vi "EMS Setpoint Status.vi"(4 "Status":T1, 6 "Error String":string, 8 "error in (no error)":errorcluster, 9 "Variable Name":string, 10 "IED Name":string, 11 "Master Controller in":refnum<class "Master Controller.lvclass">) -> (0 "error out":errorcluster, 3 "Master Controller out":refnum<class "Master Controller.lvclass">)   [LabVIEW 2015, in "Master Controller Core.lvlib" / "Master Controller.lvclass"]
uses:
  Master Controller.lvclass
  SCADA Core/SCADA Abstract Messages/IED Setpoint Status Msg/IED Setpoint Status.ctl
  Communications/SCADA Communcations Actor/SCADA Communications/Controls/EMS Message Cluster.ctl
  Master Controller.lvclass/Master Controller.ctl
  Communications/SCADA Communcations Actor/SCADA Communications Messages/Transmit EMS Message Msg/Transmit EMS Message Msg.lvclass/Transmit EMS Message Msg.ctl
  <vilib>/ActorFramework/Message Enqueuer/Message Enqueuer.lvclass/Message Enqueuer.ctl
  <vilib>/ActorFramework/Message Enqueuer/Enqueue.vi
  <vilib>/ActorFramework/Message Priority Queue/Priority Enqueue.vi
  Communications/SCADA Communcations Actor/SCADA Communications Messages/Transmit EMS Message Msg/Transmit EMS Message Msg.lvclass
  Utilities/Message Strings.llb/Message String Utilities.lvlib
  Communications/SCADA Communcations Actor/SCADA Communications/SCADA Communications.lvclass
  SCADA Core/SCADA Abstract Messages/IED Setpoint Status Msg/IED Setpoint Status Msg.lvclass
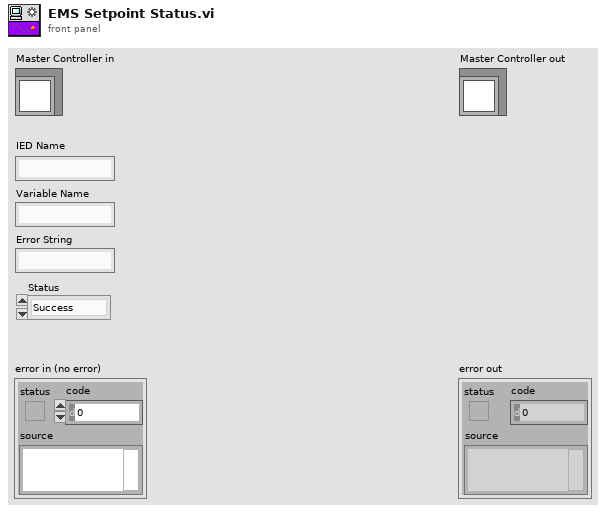
[diagram p1: front panel]
types:
  T1 = typedef "SCADA Core.lvlib/IED Setpoint Status Msg.lvclass/IED Setpoint Status.ctl" = enum16{"Success", "Failure", "Multiple Success", "Multiple Failure"}
  T2 = typedef "SCADA Communcations Actor.lvlib/SCADA Communications.lvclass/EMS Message Cluster.ctl" = cluster{"Name":string, "Content":string}
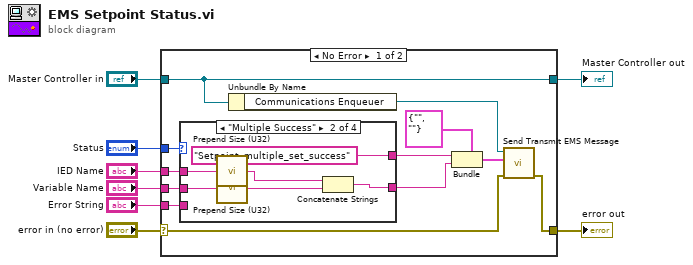
[diagram p0: block diagram]
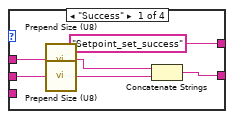
[diagram p2: hidden frame]
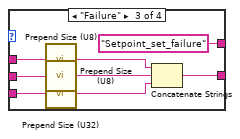
[diagram p3: hidden frame]
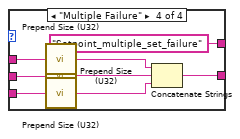
[diagram p4: hidden frame]
diagram:
  n1 = case shown="No Error" "error in (no error)" {
    selector: "error in (no error)" -> [w14 w50]
    tunnel: [w9 w50] -> w7
    tunnel: [w15 w49] -> w5
    tunnel: "Master Controller in" -> [w15 w49]
    tunnel: "Status" -> [w13 _]
    tunnel: "IED Name" -> [w12 _]
    tunnel: "Variable Name" -> [w11 _]
    tunnel: "Error String" -> [w10 _]
    frame No Error {
      n2 = case shown="\"Multiple Success\"" w13 {
        tunnel: ["Setpoint_set_success" ("Name") "Setpoint_multiple_set_success" ("Name") "Setpoint_set_failure" ("Name") "Setpoint_multiple_set_failure" ("Name")] -> w19
        tunnel: w10 -> [_ _ w38 w46]
        tunnel: w11 -> [w25 w31 w39 w47]
        tunnel: w12 -> [w24 w30 w37 w45]
        tunnel: [w21 w27 w33 w41] -> w20
        frame "Success" {
          n3 = call "Prepend Size (U8).vi"("String in"=w24) -> ("String out"=w23:string)
          n4 = call "Prepend Size (U8).vi"("String in"=w25) -> ("String out"=w22:string)
          n5 = Concatenate Strings(w23, w22) -> (w21:string)
        }
        frame "Multiple Success" {
          n6 = call "Prepend Size (U32).vi"("String in"=w30) -> ("String out"=w29:string)
          n7 = call "Prepend Size (U32).vi"("String in"=w31) -> ("String out"=w28:string)
          n8 = Concatenate Strings(w29, w28) -> (w27:string)
        }
        frame "Failure" {
          n9 = call "Prepend Size (U8).vi"("String in"=w37) -> ("String out"=w35:string)
          n10 = call "Prepend Size (U8).vi"("String in"=w39) -> ("String out"=w36:string)
          n11 = call "Prepend Size (U32).vi"("String in"=w38) -> ("String out"=w34:string)
          n12 = Concatenate Strings(w35, w36, w34) -> (w33:string)
        }
        frame "Multiple Failure" {
          n13 = call "Prepend Size (U32).vi"("String in"=w45) -> ("String out"=w43:string)
          n14 = call "Prepend Size (U32).vi"("String in"=w47) -> ("String out"=w44:string)
          n15 = call "Prepend Size (U32).vi"("String in"=w46) -> ("String out"=w42:string)
          n16 = Concatenate Strings(w43, w44, w42) -> (w41:string)
        }
      }
      n17 = Unbundle By Name(w15) -> ("Communications Enqueuer"=w17:refnum<class "Message Enqueuer.lvclass">)
      n18 = Bundle(cluster=T2 {"Name"="", "Content"=""} ("Message"), "Name"=w19, "Content"=w20) -> (w18:T2)
      n19 = call "Send Transmit EMS Message.vi"("error in (no error)"=w14, "Message"=w18, "Message Enqueuer"=w17) -> ("error out"=w9:errorcluster)  [unwired: 7 in, 1 out]
    }
    frame Error {
    }
  }
  "error out" <- w7
  "Master Controller out" <- w5
